vi "2023_day16 (SubVI Calculate Beam Path).vi"(11 "Beam in":T1={"Map"=[], "Direction"=enum."UP", "Position (Row,Col)"=[], "Energized Tiles"=[]}) -> (3 "Beam out":T1={"Map"=[], "Direction"=enum."UP", "Position (Row,Col)"=[], "Energized Tiles"=[]})   [LabVIEW 2021]
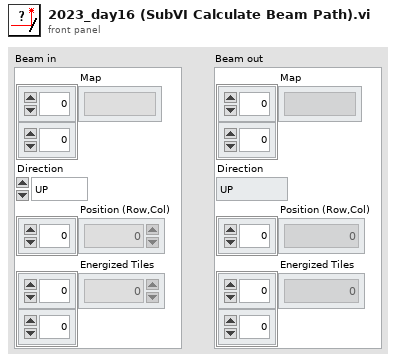
[diagram p1: front panel]
types:
  T1 = cluster{"Map":string[][], "Direction":enum16{"UP", "LEFT", "DOWN", "RIGHT"}, "Position (Row,Col)":i32[], "Energized Tiles":i32[][]}
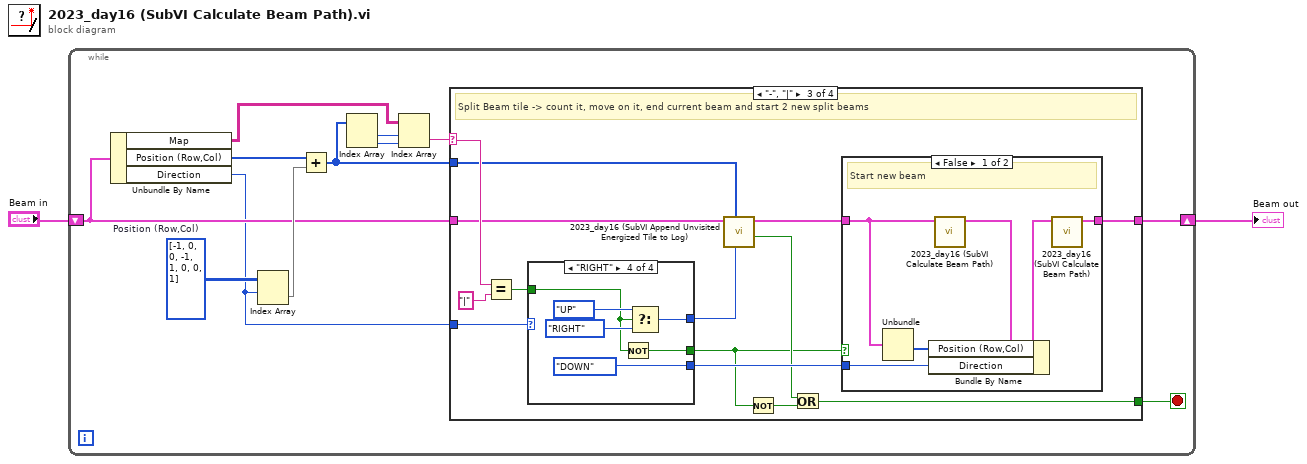
[diagram p0: block diagram]
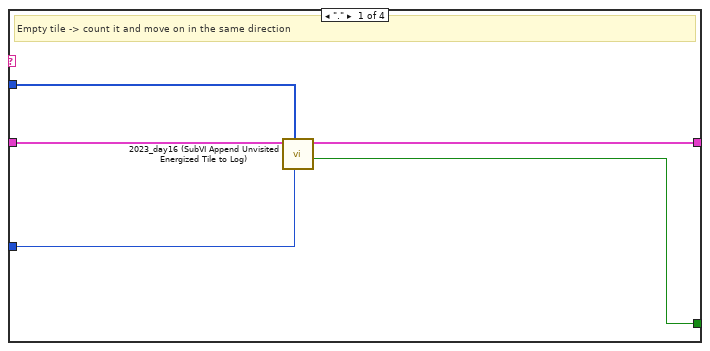
[diagram p2: hidden frame]
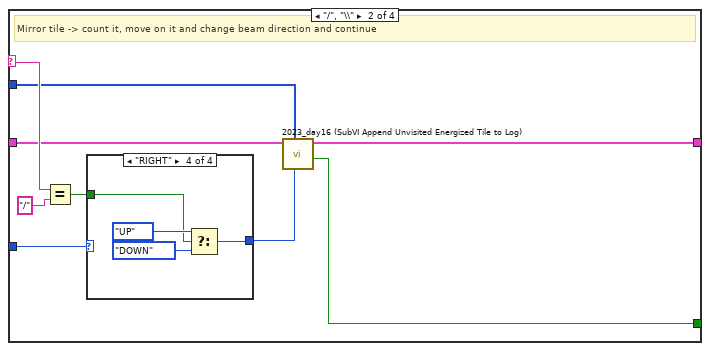
[diagram p3: hidden frame]
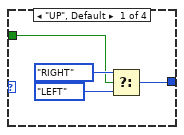
[diagram p4: hidden frame]
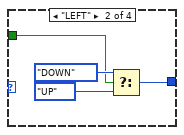
[diagram p5: hidden frame]
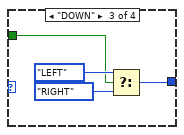
[diagram p6: hidden frame]
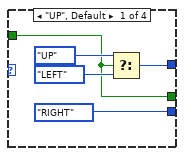
[diagram p7: hidden frame]
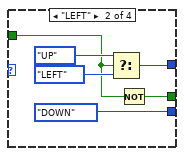
[diagram p8: hidden frame]
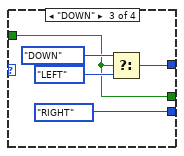
[diagram p9: hidden frame]
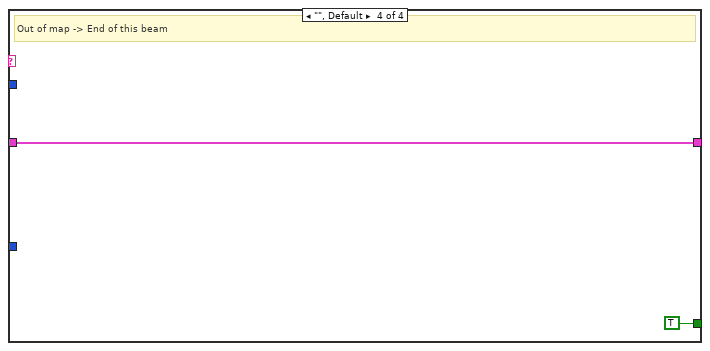
[diagram p11: hidden frame]
diagram:
  n1 = while {
    shift-right: [w7] -> w2
    shift-left: "Beam in" -> [w10]
    stop <- w8 stop-if-true
    w14 = i32[][] [[-1, 0], [0, -1], [1, 0], [0, 1]]  # Position (Row,Col)
    n2 = Unbundle By Name(w10) -> ("Map"=w4:string[][], "Position (Row,Col)"=w3:i32[], "Direction"=w5:enum16{"UP", "LEFT", "DOWN", "RIGHT"})
    n3 = Index Array(array=w14, index (row)=w5) -> (element=w13:i32[])  [unwired: 1 in]
    n4 = Add(x=w3, y=w13) -> (x+y=w6:i32[])
    n5 = Index Array(array=w6) -> (element #1=w12:i32, element #2=w11:i32)  [unwired: 2 in]
    n6 = Index Array(array=w4, index (row)=w12, index (col)=w11) -> (element=w9:string)
    n7 = case shown="\"-\", \"|\"" w9 {
      selector: w9 -> [_ w24 w56 _]
      tunnel: [w15 w20 w50 TRUE] -> w8
      tunnel: w10 -> [w19 w23 w53 w88]
      tunnel: [w18 w28 w54 w88] -> w7
      tunnel: w6 -> [w16 w22 w52 _]
      tunnel: w5 -> [w17 w27 w48 _]
      frame "." {
        # "Empty tile -> count it and move on in the same direction"
        n8 = call "2023_day16 (SubVI Append Unvisited Energized Tile to Log).vi"("Next Direction"=w17, "Next Position (Row,Col)"=w16, "Beam in"=w19) -> ("Stop"=w15:bool, "Beam out"=w18:T1)  [unwired: 7 in]
      }
      frame "/", "\\" {
        # "Mirror tile -> count it, move on it and change beam direction and continue"
        n9 = Equal?(x=w24, y="/" ("x")) -> (x = y?=w25:bool)
        n10 = case shown="\"RIGHT\"" w27 {
          tunnel: [w30 w34 w38 w42] -> w21
          tunnel: w25 -> [w29 w33 w37 w41]
          frame "UP", Default {
            n11 = Select(t=enum16{"UP", "LEFT", "DOWN", "RIGHT"}."RIGHT" ("Direction"), s=w29, f=enum16{"UP", "LEFT", "DOWN", "RIGHT"}."LEFT" ("Direction")) -> (s? t:f=w30:enum16{"UP", "LEFT", "DOWN", "RIGHT"})
          }
          frame "LEFT" {
            n12 = Select(t=enum16{"UP", "LEFT", "DOWN", "RIGHT"}."DOWN" ("Direction"), s=w33, f=enum16{"UP", "LEFT", "DOWN", "RIGHT"}."UP" ("Direction")) -> (s? t:f=w34:enum16{"UP", "LEFT", "DOWN", "RIGHT"})
          }
          frame "DOWN" {
            n13 = Select(t=enum16{"UP", "LEFT", "DOWN", "RIGHT"}."LEFT" ("Direction"), s=w37, f=enum16{"UP", "LEFT", "DOWN", "RIGHT"}."RIGHT" ("Direction")) -> (s? t:f=w38:enum16{"UP", "LEFT", "DOWN", "RIGHT"})
          }
          frame "RIGHT" {
            n14 = Select(t=enum16{"UP", "LEFT", "DOWN", "RIGHT"}."UP" ("Direction"), s=w41, f=enum16{"UP", "LEFT", "DOWN", "RIGHT"}."DOWN" ("Direction")) -> (s? t:f=w42:enum16{"UP", "LEFT", "DOWN", "RIGHT"})
          }
        }
        n15 = call "2023_day16 (SubVI Append Unvisited Energized Tile to Log).vi"("Next Direction"=w21, "Next Position (Row,Col)"=w22, "Beam in"=w23) -> ("Stop"=w20:bool, "Beam out"=w28:T1)  [unwired: 7 in]
      }
      frame "-", "|" {
        # "Split Beam tile -> count it, move on it, end current beam and start 2 new split beams"
        n16 = Equal?(x=w56, y="|" ("x")) -> (x = y?=w57:bool)
        n17 = case shown="\"RIGHT\"" w48 {
          tunnel: [w61 w67 w72 w78] -> w45
          tunnel: w57 -> [w59 w65 w70 w76]
          tunnel: [enum16{"UP", "LEFT", "DOWN", "RIGHT"}."RIGHT" ("Direction") enum16{"UP", "LEFT", "DOWN", "RIGHT"}."DOWN" ("Direction") enum16{"UP", "LEFT", "DOWN", "RIGHT"}."RIGHT" ("Direction") enum16{"UP", "LEFT", "DOWN", "RIGHT"}."DOWN" ("Direction")] -> w55
          tunnel: [w59 w64 w70 w75] -> w47
          frame "UP", Default {
            n18 = Select(t=enum16{"UP", "LEFT", "DOWN", "RIGHT"}."UP" ("Direction"), s=w59, f=enum16{"UP", "LEFT", "DOWN", "RIGHT"}."LEFT" ("Direction")) -> (s? t:f=w61:enum16{"UP", "LEFT", "DOWN", "RIGHT"})
          }
          frame "LEFT" {
            n19 = Select(t=enum16{"UP", "LEFT", "DOWN", "RIGHT"}."UP" ("Direction"), s=w65, f=enum16{"UP", "LEFT", "DOWN", "RIGHT"}."LEFT" ("Direction")) -> (s? t:f=w67:enum16{"UP", "LEFT", "DOWN", "RIGHT"})
            n20 = Not(x=w65) -> (.not. x?=w64:bool)
          }
          frame "DOWN" {
            n21 = Select(t=enum16{"UP", "LEFT", "DOWN", "RIGHT"}."DOWN" ("Direction"), s=w70, f=enum16{"UP", "LEFT", "DOWN", "RIGHT"}."LEFT" ("Direction")) -> (s? t:f=w72:enum16{"UP", "LEFT", "DOWN", "RIGHT"})
          }
          frame "RIGHT" {
            n22 = Not(x=w76) -> (.not. x?=w75:bool)
            n23 = Select(t=enum16{"UP", "LEFT", "DOWN", "RIGHT"}."UP" ("Direction"), s=w76, f=enum16{"UP", "LEFT", "DOWN", "RIGHT"}."RIGHT" ("Direction")) -> (s? t:f=w78:enum16{"UP", "LEFT", "DOWN", "RIGHT"})
          }
        }
        n24 = call "2023_day16 (SubVI Append Unvisited Energized Tile to Log).vi"("Next Direction"=w45, "Next Position (Row,Col)"=w52, "Beam in"=w53) -> ("Stop"=w49:bool, "Beam out"=w51:T1)  [unwired: 7 in]
        n25 = Not(x=w47) -> (.not. x?=w46:bool)
        n26 = Or(x=w49, y=w46) -> (x .or. y?=w50:bool)
        n27 = case shown="False" w47 {
          tunnel: w51 -> [w82 w87]
          tunnel: w55 -> [w83 _]
          tunnel: [w84 w87] -> w54
          frame False {
            # "Start new beam"
            n28 = Unbundle(w82) -> ("Position (Row,Col)"=w81:i32[])  [unwired: 3 out]
            n29 = call "2023_day16 (SubVI Calculate Beam Path).vi"("Beam in"=w82) -> ("Beam out"=w86:T1)  [unwired: 10 in]
            n30 = Bundle By Name(cluster=w86, "Position (Row,Col)"=w81, "Direction"=w83) -> (w85:T1)
            n31 = call "2023_day16 (SubVI Calculate Beam Path).vi"("Beam in"=w85) -> ("Beam out"=w84:T1)  [unwired: 10 in]
          }
          frame True {
            # "Continue Single Beam"
          }
        }
      }
      frame "", Default {
        # "Out of map -> End of this beam"
      }
    }
  }
  "Beam out" <- w2
